vi "DigSeqLogic_Delay.vi"(8 "Time":dbl=-1.0, 9 "Delay Time":dbl=1.0, 11 "Input":bool) -> (1 "IsPresent":bool, 3 "Output":bool)   [LabVIEW 2019, in "Trajectory_Library.lvlib"]
doc: "This VI implements a digital \"time delay\". The output is the input delayed by \"Delay\" seconds. If the \"Delay\" time does not exactly match the sample period, the boolean value prior to the delay time is returned.\n\nInputs:\n - Input -- Boolean input value\n - Delay Time -- Time (seconds) to delay the otuput value. If time delay is increaed, then the buffer is re-created. FALSE will be returned until the buffer has sufficient data to return a delayed value.\n - Time -- Continously counting system time, Seconds. If not wired the FPGA time will be used.\n\nOutputs:\n - Output -- Boolean output value with delay applied\n - IsPresent -- Set to TRUE if the buffer has enough data to return a delayed value."
uses:
  Trajectory_Library.lvlib
  TimeInterpBoolean_CleanUp.vi
  <vilib>/gmath/interp.llb/Search Ordered Table.vi
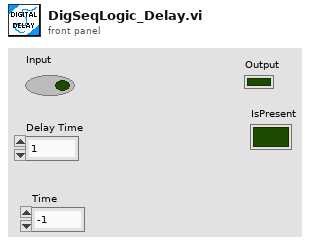
[diagram p1: front panel]
types:
  T1 = typedef "Trajectory_Library.lvlib/TIME_INTERPOLATABLE_BOOLEAN.ctl" = cluster{"TimeStamps":dbl[], "BooleanValue":bool[], "Min_TimeStamp":dbl, "Max_TimeStamp":dbl, "ItemCount":i32, "MaxBufferTime":dbl}
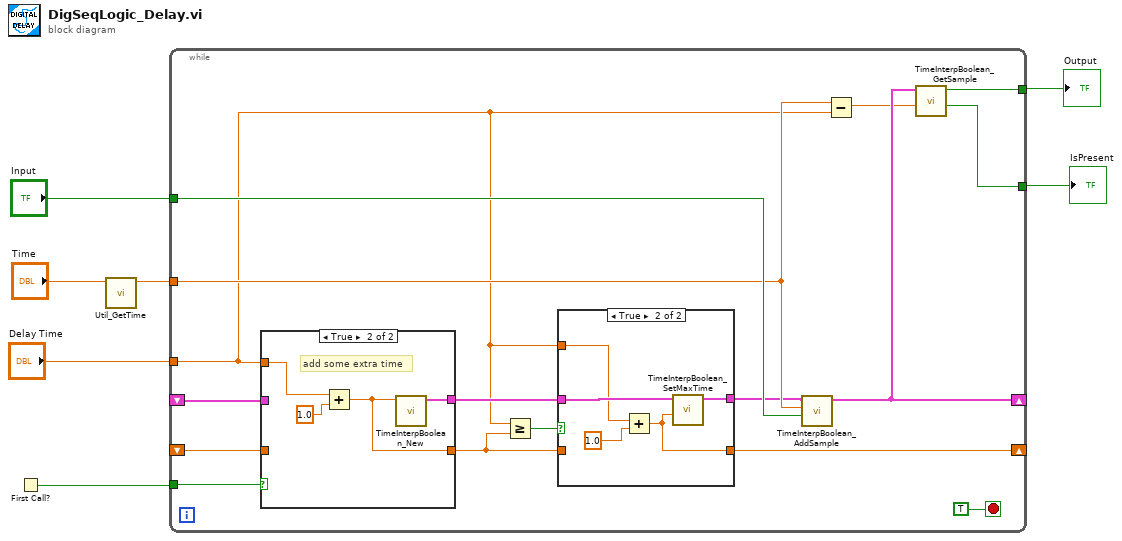
[diagram p0: block diagram]
diagram:
  n1 = First Call?() -> (First Call?: T/F=w6:bool)
  n2 = call "Util_GetTime.vi"("Pass_Through_Time"="Time") -> ("FPGA_Time_Seconds"=w4:dbl)  [unwired: 9 in, 1 out]
  n3 = while {
    tunnel: "Delay Time" -> [w11]
    tunnel: w6 -> [w14]
    shift-right: [w21] -> _
    shift-left: _ -> [w16]
    tunnel: w4 -> [w20]
    tunnel: "Input" -> [w22]
    tunnel: [w18] -> w2
    tunnel: [w17] -> w1
    shift-right: [w9] -> _
    shift-left: _ -> [w15]
    stop <- TRUE stop-if-true
    n4 = case shown="True" w14 {
      tunnel: w11 -> [_ w34]
      tunnel: [w32 w35] -> w12
      tunnel: w16 -> [w32 _]
      tunnel: [w31 w33] -> w8
      tunnel: w15 -> [w31 _]
      frame False {
      }
      frame True {
        # "add some extra time"
        n5 = Add(x=w34, y=1.0) -> (x+y=w33:dbl)
        n6 = call "TimeInterpBoolean_New.vi"("MaxTime"=w33) -> ("TimeInterpBoolean"=w35:T1)  [unwired: 10 in]
      }
    }
    n7 = Greater Or Equal?(x=w11, y=w8) -> (x >= y?=w13:bool)
    n8 = case shown="True" w13 {
      tunnel: w12 -> [w25 w30]
      tunnel: w11 -> [_ w28]
      tunnel: [w25 w27] -> w10
      tunnel: [w24 w26] -> w9
      tunnel: w8 -> [w24 _]
      frame False {
      }
      frame True {
        n9 = Add(x=w28, y=1.0) -> (x+y=w26:dbl)
        n10 = call "TimeInterpBoolean_SetMaxTime.vi"("Max Time"=w26, "in TimeInterpBoolean"=w30) -> ("out TimeInterpBoolean"=w27:T1)  [unwired: 9 in]
      }
    }
    n11 = call "TimeInterpBoolean_AddSample.vi"("Value"=w22, "TimeStamp"=w20, "in TimeInterpBoolean"=w10) -> ("out TimeInterpBoolean"=w21:T1)  [unwired: 7 in, 1 out]
    n12 = Subtract(x=w20, y=w11) -> (x-y=w19:dbl)
    n13 = call "TimeInterpBoolean_GetSample.vi"("TimeStamp"=w19, "TimeInterpBoolean"=w21) -> ("IsPresent"=w17:bool, "OutputBoolean"=w18:bool)  [unwired: 8 in]
  }
  "Output" <- w2
  "IsPresent" <- w1
